vi "Deg-Ft 6in Mecanum.vi"(5 "Input":dbl) -> (2 "Output":dbl)   [LabVIEW 2014]
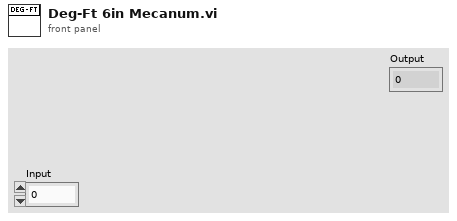
[diagram p1: front panel]
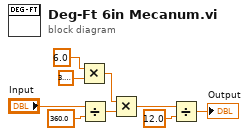
[diagram p0: block diagram]
diagram:
  n1 = Multiply(x=6.0, y=3.141592653589793) -> (x*y=w7:dbl)
  n2 = Divide(x="Input", y=360.0) -> (x/y=w4:dbl)
  n3 = Multiply(x=w7, y=w4) -> (x*y=w6:dbl)
  n4 = Divide(x=w6, y=12.0) -> (x/y=→"Output":dbl)
